vi "Calcul itératif.vi"(8 "error in (no error)":T1 caption="entrée d'erreur (pas d'erreur)", 10 "Température capteur 1-2-3-4-Ambiant":dbl[](array[numeric]), 11 "Position des capteurs":dbl[][](array[numeric])) -> (0 "error out":T1 caption="sortie d'erreur", 3 "DATA - T/R1/R2/R3":dbl[](array[numeric]) format="%#_13g")   [LabVIEW 2018]
panel:
  in  "T max":dbl
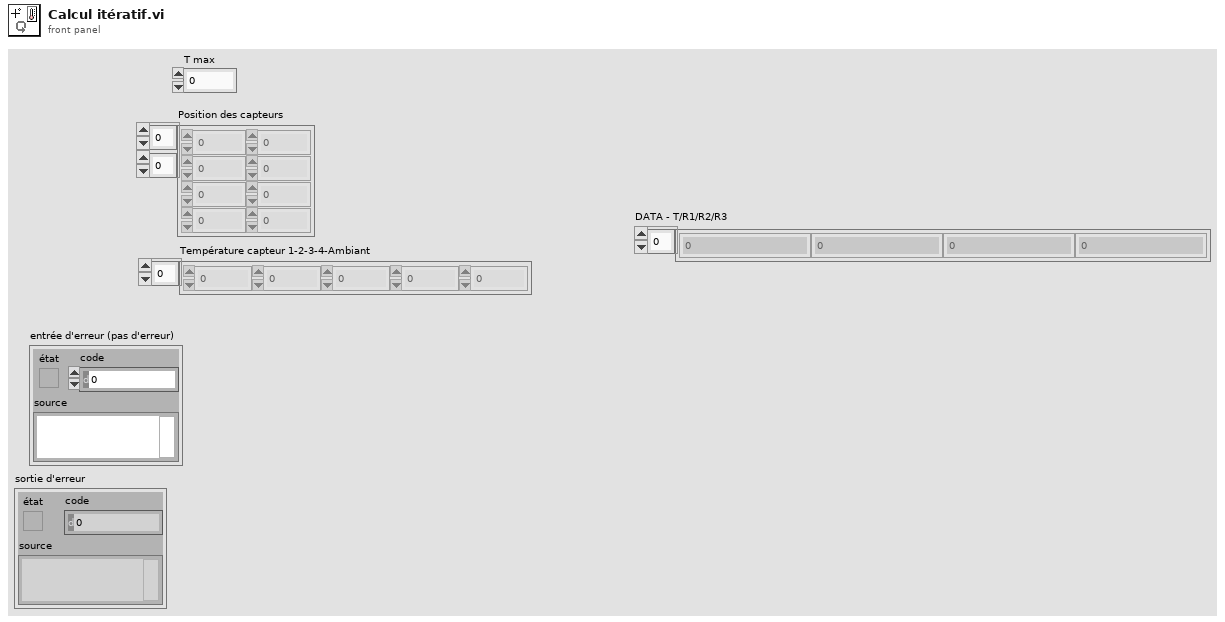
[diagram p1: front panel]
types:
  T1 = cluster{"état":bool, "code":i32, "source":string}
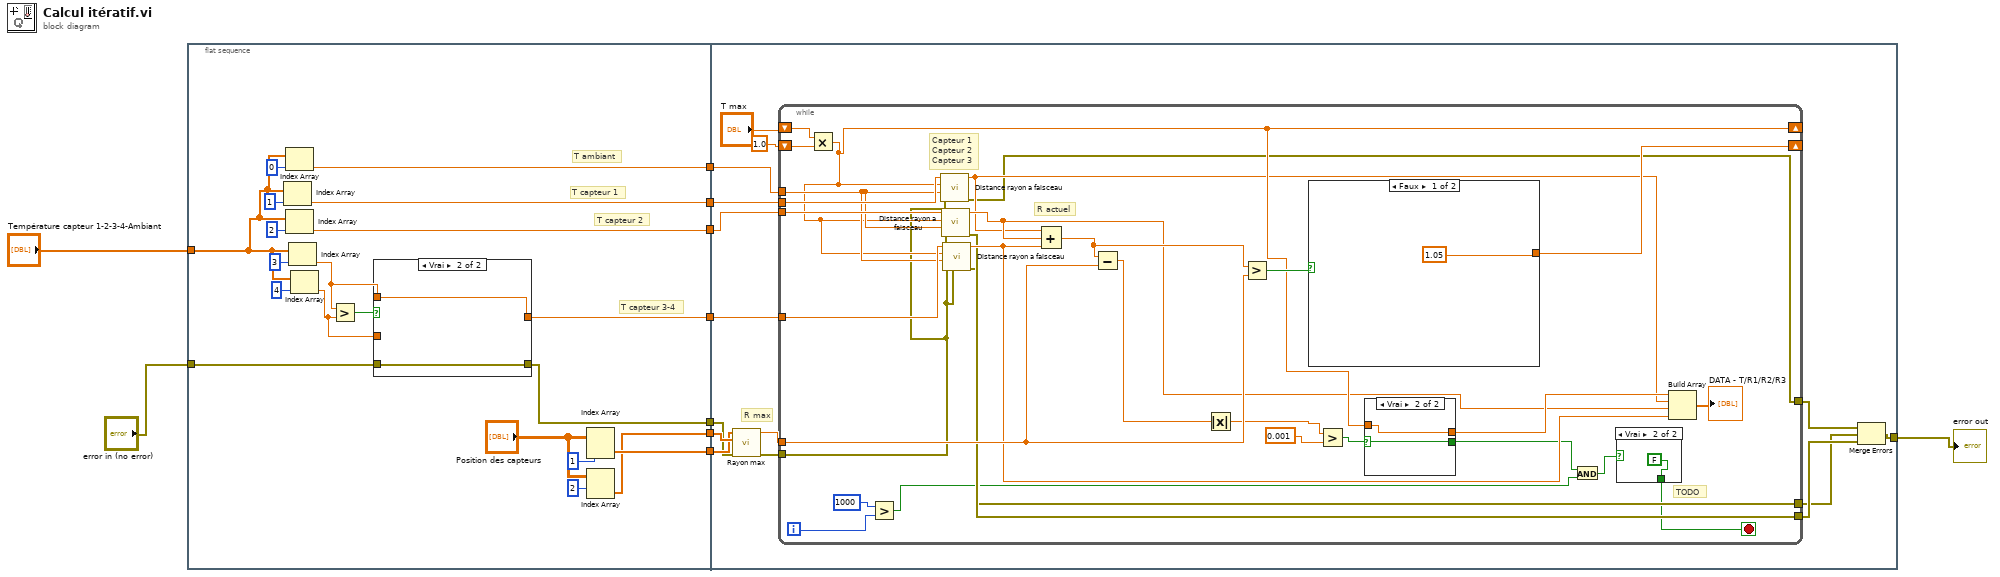
[diagram p0: block diagram]
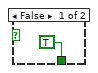
[diagram p3: hidden frame]
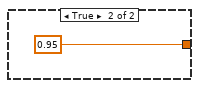
[diagram p5: hidden frame]
diagram:
  n1 = flat-sequence {
    tunnel: "Température capteur 1-2-3-4-Ambiant" -> [w20]
    tunnel: [w26] -> w10
    tunnel: [w22] -> w9
    tunnel: [w21] -> w8
    tunnel: [w18] -> w7
    tunnel: [w14] -> w5
    tunnel: [w13] -> w4
    tunnel: "error in (no error)" -> [w12]
    tunnel: [w11] -> w2
    tunnel: w10 -> [w46]
    tunnel: w9 -> [w49]
    tunnel: w8 -> [w47]
    tunnel: w7 -> [w48]
    tunnel: w5 -> [w42]
    tunnel: w4 -> [w43]
    tunnel: w2 -> [w40]
    tunnel: [w35] -> w1
    frame #0 {
      # "T capteur 3-4"
      # "T capteur 2"
      # "T capteur 1"
      # "T ambiant"
      n2 = Index Array(array=w20, index=1 ("indice")) -> (element=w22:dbl)
      n3 = Index Array(array=w20, index=0 ("indice")) -> (element=w18:dbl)
      n4 = Index Array(array=w20, index=2 ("indice")) -> (element=w21:dbl)
      n5 = Index Array(array=w20, index=3 ("indice")) -> (element=w27:dbl)
      n6 = Index Array(array=w20, index=4 ("indice")) -> (element=w25:dbl)
      n7 = Greater?(x=w27, y=w25) -> (0:w28:bool)
      n8 = case shown="Vrai" w28 {
        tunnel: [w32 w34] -> w26
        tunnel: w27 -> [_ w34]
        tunnel: w25 -> [w32 _]
        tunnel: w12 -> [w31 w33]
        tunnel: [w31 w33] -> w11
        frame False {
        }
        frame True {
        }
      }
      n9 = Index Array(array="Position des capteurs", index (row)=1 ("indice (ligne)")) -> (element=w14:dbl[])  [unwired: 1 in]
      n10 = Index Array(array="Position des capteurs", index (row)=2 ("indice (ligne)")) -> (element=w13:dbl[])  [unwired: 1 in]
    }
    frame #1 {
      # "R max"
      n11 = call "Rayon max.vi"("error in (no error)"=w40, "Capteur 3 ou 4"=w43, "Capteur 2"=w42) -> ("error out"=w39:T1, "Rayon max"=w41:dbl)  [unwired: 7 in]
      n12 = while {
        tunnel: w49 -> [w79]
        tunnel: w48 -> [w76]
        tunnel: w47 -> [w78]
        tunnel: w46 -> [w77]
        shift-right: [w73] -> _
        shift-left: 1.0 -> [w71]
        shift-right: [w68] -> _
        shift-left: "T max" -> [w70]
        tunnel: w41 -> [w69]
        tunnel: w39 -> [w62]
        tunnel: [w61] -> w36
        tunnel: [w60] -> w38
        tunnel: [w59] -> w37
        i -> [w54]
        stop <- w50 stop-if-true
        # "Capteur 1\nCapteur 2\nCapteur 3"
        # "R actuel"
        # "TODO"
        n13 = Multiply(x=w70, y=w71) -> (x*y=w68:dbl)
        n14 = Greater?(x=1000, y=w54) -> (0:w52:bool)
        n15 = call "Distance rayon a faisceau.vi"("error in (no error)"=w62, "T ambiant"=w76, "T max"=w68, "T capteur"=w79) -> ("error out"=w61:T1, "Rayon"=w63:dbl)  [unwired: 6 in]
        n16 = call "Distance rayon a faisceau.vi"("error in (no error)"=w62, "T ambiant"=w76, "T max"=w68, "T capteur"=w78) -> ("error out"=w60:T1, "Rayon"=w66:dbl)  [unwired: 6 in]
        n17 = call "Distance rayon a faisceau.vi"("error in (no error)"=w62, "T ambiant"=w76, "T max"=w68, "T capteur"=w77) -> ("error out"=w59:T1, "Rayon"=w65:dbl)  [unwired: 6 in]
        n18 = Compound Arithmetic op=ADD(w63, w66, w65) -> (w74:dbl)
        n19 = Subtract(x=w74, y=w69) -> (x-y=w75:dbl)
        n20 = Absolute Value(x=w75) -> (abs(x)=w57:dbl)
        n21 = Greater?(x=w74, y=w69) -> (0:w72:bool)
        n22 = case shown="Faux" w72 {
          tunnel: [1.05 0.95] -> w73
          frame False {
          }
          frame True {
          }
        }
        n23 = Greater?(x=w57, y=0.001) -> (0:w55:bool)
        n24 = case shown="Vrai" w55 {
          selector: w55 -> [w82 w84]
          tunnel: w68 -> [w83 w85]
          tunnel: [w83 w85] -> w67
          tunnel: [w82 w84] -> w58
          frame False {
          }
          frame True {
          }
        }
        n25 = And(x=w58, y=w52) -> (x .and. y?=w51:bool)
        n26 = case shown="Vrai" w51 {
          tunnel: [TRUE FALSE] -> w50
          frame False {
          }
          frame True {
          }
        }
        n27 = Build Array(w67, w63, w66, w65) -> (→"DATA - T/R1/R2/R3":dbl[])
      }
      n28 = Merge Errors(w36, w37, w38) -> (w35:errorcluster)
    }
  }
  "error out" <- w1
